vi "get result path start.vi"(0 "main VI path":path) -> (4 "result file path":path)   [LabVIEW 2019]
doc: "This subVI uses the main VI's path as a reference pointer to choose the result data file path."
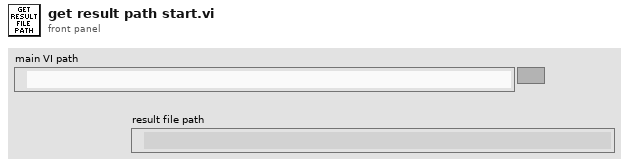
[diagram p1: front panel]
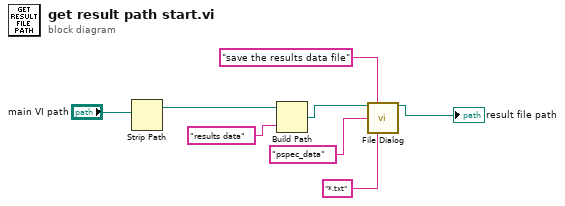
[diagram p0: block diagram]
diagram:
  n1 = Strip Path(path="main VI path") -> (stripped path=w7:path)  [unwired: 1 out]
  n2 = Build Path(base path=w7, name or relative path="results data") -> (appended path=w6:path)
  n3 = call "File Dialog"("start path"=w6, "prompt"="save the results data file", "default name"="pspec_data", "pattern (all files)"="*.txt") -> ("selected path"=→"result file path":path)  [unwired: 8 in, 3 out]
